vi "Configure Arbitrary Waveform Data.vi"(6 "Waveform Generator Number (1: Waveform Generator 1)":i32(ring)=1 items=["Waveform Generator 1"=1, "Waveform Generator 2"=2], 7 "16-bit Integer Data":i32[](array[numeric])=[0], 8 "error in (no error)":errorcluster, 9 "Floating-Point Data":dbl[](array[numeric])=[0.0], 10 "Data Format (0: Floating Point Value)":i32(ring) items=["Floating Point Value", "16-bit Integer Value"], 11 "VISA resource name":refnum<visa-resource-name>) -> (0 "error out":errorcluster, 3 "VISA resource name out":refnum<visa-resource-name>)   [LabVIEW 2015, in "Agilent 2000 3000 X-Series.lvlib"]
doc: "Configures the arbitrary waveform data."
uses:
  <instrlib>/Agilent 2000 3000 X-Series/Agilent 2000 3000 X-Series.lvlib
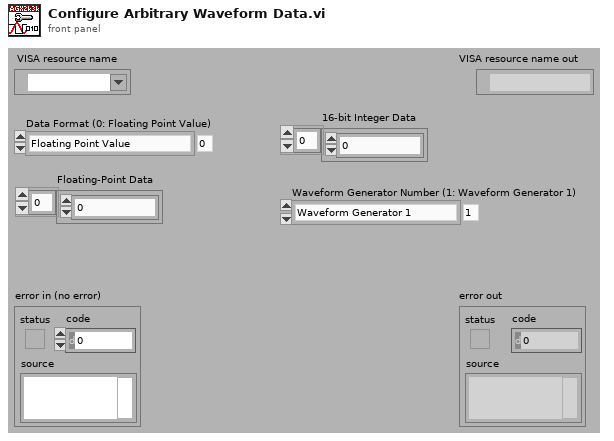
[diagram p1: front panel]
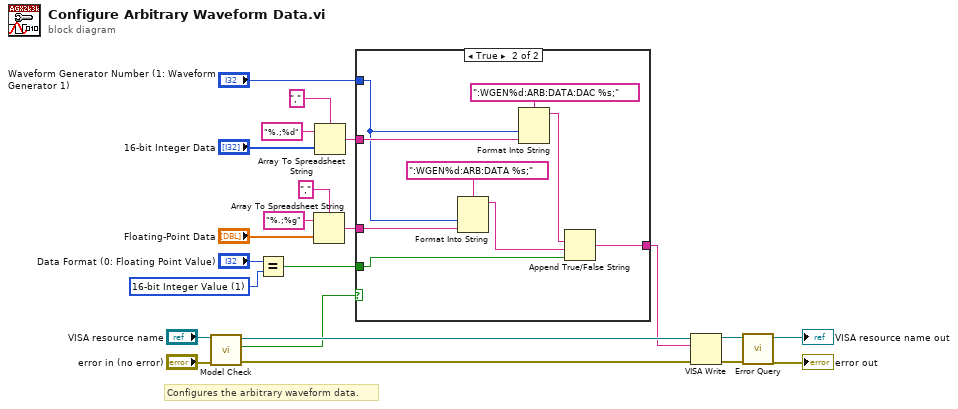
[diagram p0: block diagram]
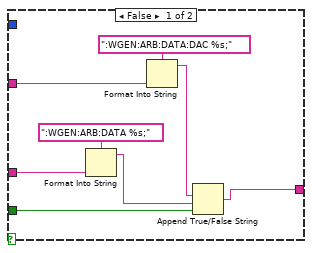
[diagram p2: hidden frame]
diagram:
  w2 = 1 items=["Floating Point Value", "16-bit Integer Value"] ("Data Format (0: Floating Point Value)")
  # "Configures the arbitrary waveform data."
  n1 = call <instrlib>:"Model Check.vi"("error in (no error)"="error in (no error)", "VISA resource name"="VISA resource name") -> ("error out"=w11:errorcluster, "Not 2000 or 3000 Series"=w8:bool, "VISA resource name out"=w12:refnum<visa-resource-name>)  [unwired: 7 out]
  n2 = Equal?(x="Data Format (0: Floating Point Value)", y=w2) -> (x = y?=w1:bool)
  n3 = Array To Spreadsheet String(delimiter (Tab)=",", array="Floating-Point Data", 3:"%.;%g" ("format string")) -> (spreadsheet string=w9:string)
  n4 = Array To Spreadsheet String(delimiter (Tab)=",", array="16-bit Integer Data", 3:"%.;%d" ("format string")) -> (spreadsheet string=w10:string)
  n5 = case shown="True" w8 {
    tunnel: w10 -> [w26 w35]
    tunnel: w9 -> [w25 w32]
    tunnel: w1 -> [w24 w31]
    tunnel: [w23 w34] -> w7
    tunnel: "Waveform Generator Number (1: Waveform Generator 1)" -> [_ w33]
    frame False {
      n6 = Format Into String(format string=":WGEN:ARB:DATA %s;", w25) -> (resulting string=w27:string)  [unwired: 2 in, 1 out]
      n7 = Format Into String(format string=":WGEN:ARB:DATA:DAC %s;", w26) -> (resulting string=w29:string)  [unwired: 2 in, 1 out]
      n8 = Append True/False String(1:w24, 2:w27, 3:w29) -> (0:w23:string)  [unwired: 1 out]
    }
    frame True {
      n9 = Format Into String(format string=":WGEN%d:ARB:DATA %s;", w33, w32) -> (resulting string=w36:string)  [unwired: 2 in, 1 out]
      n10 = Format Into String(format string=":WGEN%d:ARB:DATA:DAC %s;", w33, w35) -> (resulting string=w38:string)  [unwired: 2 in, 1 out]
      n11 = Append True/False String(1:w31, 2:w36, 3:w38) -> (0:w34:string)  [unwired: 1 out]
    }
  }
  n12 = VISA Write(VISA resource name=w12, write buffer=w7, error in (no error)=w11) -> (VISA resource name out=w22:refnum<visa-resource-name>, error out=w21:errorcluster)  [unwired: 1 out]
  n13 = call <instrlib>:"Error Query.vi"("error in (no error)"=w21, "VISA resource name"=w22) -> ("error out"=→"error out":errorcluster, "VISA resource name out"=→"VISA resource name out":refnum<visa-resource-name>)  [unwired: 8 out]
